vi "Test No Connection Errors.vi"() -> ()   [LabVIEW 2013]
uses:
  source/MQTT_Connection/Connection/Connection.lvclass
panel:
  out "error out 6":errorcluster
  out "error out 5":errorcluster
  out "error out 4":errorcluster
  out "error out 3":errorcluster
  out "error out 2":errorcluster
  out "error out":errorcluster
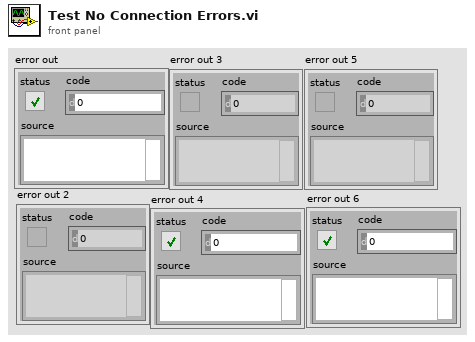
[diagram p1: front panel]
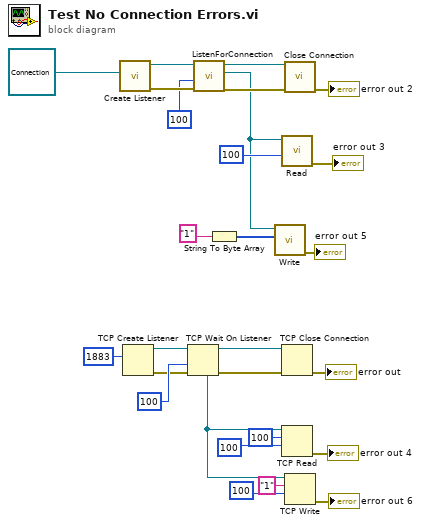
[diagram p0: block diagram]
diagram:
  n1 = call "Create Listener.vi"("Connection Configuration"=refnum<class "Connection.lvclass"> refnum ("MQTT_Connection.lvlib:Connection.lvclass")) -> ("error out"=w16:errorcluster, "Listener"=w27:refnum<class "Connection.lvclass">)  [unwired: 9 in]
  n2 = TCP Create Listener(10:u16 1883 ("port")) -> (0:w20:errorcluster, 3:w23:refnum<k5>)  [unwired: 4 in, 1 out]
  n3 = TCP Wait On Listener(8:w20, 9:100 ("timeout ms (wait forever: -1)"), 11:w23) -> (0:w19:errorcluster, 3:w21:refnum<k5>, 4:w12:refnum<k5>)  [unwired: 1 in, 2 out]
  n4 = call "ListenForConnection.vi"("error in (no error)"=w16, "timeout (2000 ms)"=100 ("timeout ms (wait forever: -1)"), "Listener"=w27) -> ("error out"=w17:errorcluster, "Connection"=w1:refnum<class "Connection.lvclass">, "Listener out"=w25:refnum<class "Connection.lvclass">)  [unwired: 5 in, 1 out]
  n5 = String To Byte Array(string="1" ("data in")) -> (unsigned byte array=w9:u8[])
  n6 = call "Write.vi"("Bytes"=w9, "Connection in"=w1) -> ("error out"=→"error out 5":errorcluster)  [unwired: 8 in, 1 out]
  n7 = call "Read.vi"("timeout (2000 ms)"=100 ("bytes to read"), "TCPConnection in"=w1) -> ("error out"=→"error out 3":errorcluster)  [unwired: 5 in, 4 out]
  n8 = TCP Close Connection(connection ID=w21, error in (no error)=w19) -> (error out=→"error out":errorcluster)  [unwired: 1 in, 1 out]
  n9 = TCP Read(connection ID=w12, bytes to read=100, 9:100 ("bytes to read")) -> (error out=→"error out 4":errorcluster)  [unwired: 2 in, 2 out]
  n10 = call "Close Connection.vi"("error in (no error)"=w17, "Connection in"=w25) -> ("error out"=→"error out 2":errorcluster)  [unwired: 8 in, 1 out]
  n11 = TCP Write(connection ID=w12, data in="1", 9:100 ("bytes to read")) -> (error out=→"error out 6":errorcluster)  [unwired: 1 in, 2 out]
